vi "Test Servo.vi"() -> ()   [LabVIEW 2013]
uses:
  <vilib>/rvi/Emulation/niFpgaSctlEmulationGetInTimedLoop.vi
  <vilib>/rvi/Emulation/niFpgaEmulationReportErrorSimple.vi
  <vilib>/rvi/Emulation/niFpgaGetClockAttributes.vi
  <vilib>/rvi/eio/common/nirviEmuTemplateMethod_errors.vi
  <vilib>/rvi/Emulation/niFpgaCriticalErrorInLSC.vi
  <vilib>/eio/EIONode/EIONode.xnode
panel:
  out "error out":errorcluster
  in  "Low":u32 caption="Count(uSec)"
  in  "High":u32 caption="Count(uSec)"
  in  "Stop":bool
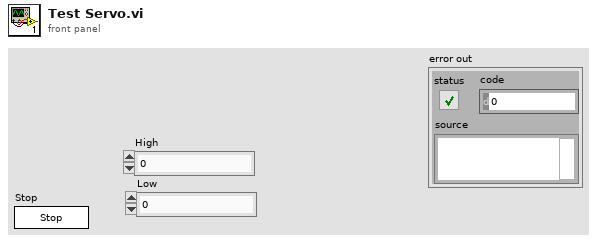
[diagram p1: front panel]
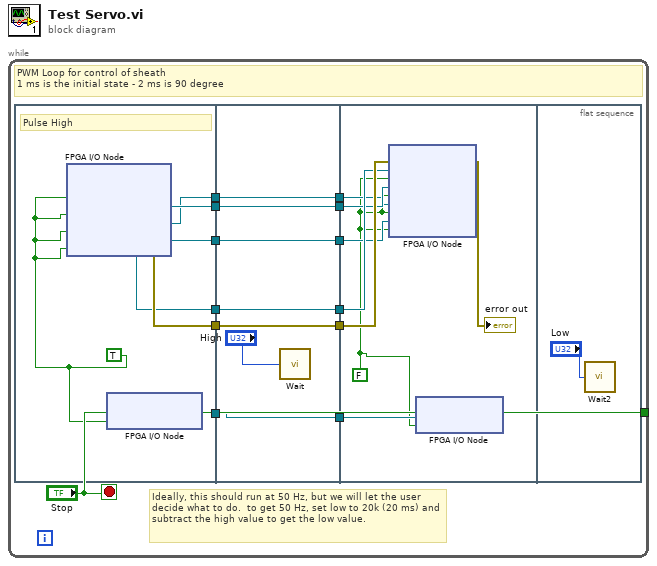
[diagram p0: block diagram]
diagram:
  n1 = while {
    tunnel: ["Stop"] -> _
    stop <- "Stop" stop-if-true
    # "Ideally, this should run at 50 Hz, but we will let the user decide what to do.  to get 50 Hz, set low to 20k (20 ms) and subtract the high value to get the low value."
    # "PWM Loop for control of sheath\n1 ms is the initial state - 2 ms is 90 degree"
    n2 = flat-sequence {
      tunnel: [w20] -> w11
      tunnel: [w19] -> w9
      tunnel: [w18] -> w8
      tunnel: [w17] -> w5
      tunnel: [w16] -> w3
      tunnel: [w15] -> w1
      tunnel: [w26] -> w12
      tunnel: w11 -> [w26]
      tunnel: [w25] -> w10
      tunnel: w9 -> [w25]
      tunnel: w8 -> [w24]
      tunnel: [w24] -> w7
      tunnel: [w23] -> w6
      tunnel: w5 -> [w23]
      tunnel: [w22] -> w4
      tunnel: w3 -> [w22]
      tunnel: [w21] -> w2
      tunnel: w1 -> [w21]
      tunnel: w12 -> [w35]
      tunnel: w10 -> [w33]
      tunnel: w7 -> [w32]
      tunnel: w6 -> [w31]
      tunnel: w4 -> [w30]
      tunnel: w2 -> [w29]
      frame #0 {
        w14 = TRUE ("Mod4/DIO0")
        # "Pulse High"
        n3 = xnode "FPGA I/O Node"("Servo PWM"=w14, "Laser Mod"=w14, "DIO2"=w14, "DIO3"=w14) -> ("error out"=w20:errorcluster, "FPGA I/O Out"=w19:refnum<k21>, "FPGA I/O Out"=w17:refnum<k21>, "FPGA I/O Out"=w16:refnum<k21>, "FPGA I/O Out"=w15:refnum<k21>)  [unwired: 5 in]
        n4 = xnode "FPGA I/O Node"("FPGA LED"=w14) -> ("FPGA I/O Out"=w18:refnum<k21>)  [unwired: 1 in]
      }
      frame #1 {
        n5 = call "Wait"("Count(uSec)"="High") -> ()  [unwired: 1 out]
      }
      frame #2 {
        w28 = FALSE ("Mod4/DIO0")
        n6 = xnode "FPGA I/O Node"("error in"=w35, "I/O Item"=w28, "FPGA I/O In"=w33, "I/O Item"=w28, "FPGA I/O In"=w31, "I/O Item"=w28, "FPGA I/O In"=w30, "I/O Item"=w28, "FPGA I/O In"=w29) -> ("error out"=→"error out":errorcluster)  [unwired: 4 out]
        n7 = xnode "FPGA I/O Node"("I/O Item"=w28, "FPGA I/O In"=w32) -> ()  [unwired: 1 out]
      }
      frame #3 {
        n8 = call "Wait2"("Count(uSec)"="Low") -> ()  [unwired: 1 out]
      }
    }
  }
